vi "MH_ReadFiFoV2.vi"(8 "error in (no error)":errorcluster, 11 "devidx":i32) -> (0 "error out":errorcluster, 1 "nactual":i32, 2 "buffer":u32[](array[numeric]), 3 "return type":i32)   [LabVIEW 2019]
uses:
  <userlib>/MultiHarp150/MH_DllPath_global.vi
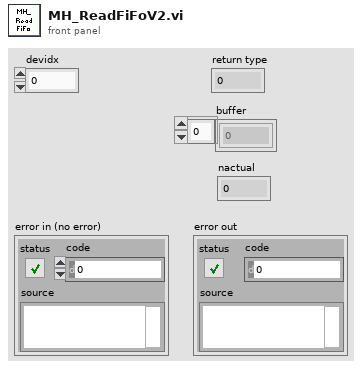
[diagram p1: front panel]
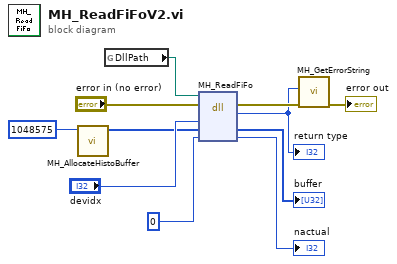
[diagram p0: block diagram]
diagram:
  n1 = call <userlib>:"MH_AllocateHistoBuffer.vi"("HistoLength"=1048575) -> ("Buffer"=w1:u32[])  [unwired: 10 in]
  n2 = global read "MH_DllPath_global.vi" "DllPath"() -> (w10:path)
  n3 = dll-call lib="MHLib64.dll" fn="MH_ReadFiFo"(path in=w10, error in="error in (no error)", "devidx"="devidx", "buffer"=w1, "nactual"=0) -> (error out=w8:errorcluster, "return type"=w7:i32, "buffer"=→"buffer":u32[], "nactual"=→"nactual":i32)  [unwired: 2 in, 1 out]
  "return type" <- w7
  n4 = call <userlib>:"MH_GetErrorString.vi"("error in (no error)"=w8, "code"=w7) -> ("error out"=→"error out":errorcluster)  [unwired: 7 in, 2 out]
